vi "Serial-to-DTV_v1.vi"(10 "Input_U8":u8[](array[numeric])) -> (0 "mseg":u16, 2 "Data Validity Time":u16[](array[numeric]))   [LabVIEW 2017]
panel:
  out "seg":u8
  out "min":u8
  out "hora":u8
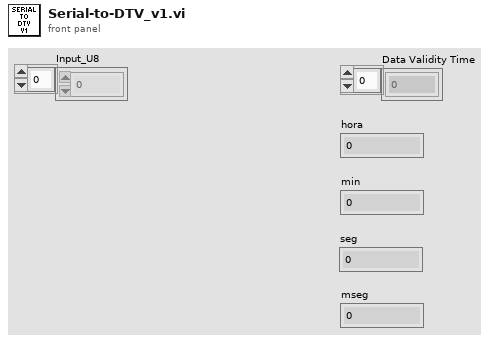
[diagram p1: front panel]
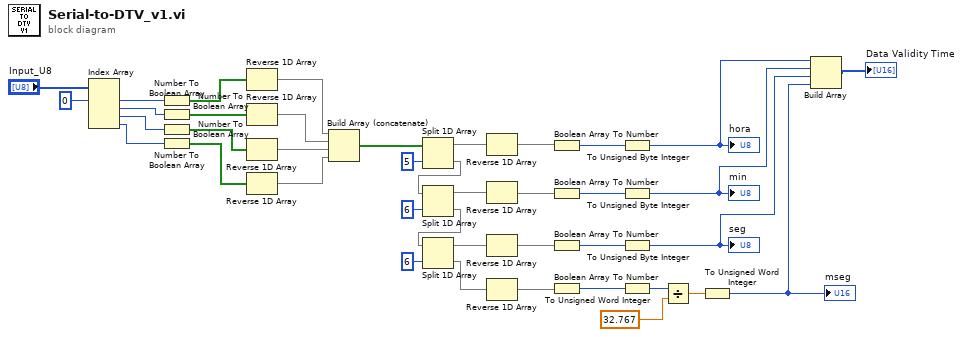
[diagram p0: block diagram]
diagram:
  n1 = Index Array(array="Input_U8", index #1=0 ("index")) -> (element #1=w36:u8, element #2=w37:u8, element #3=w38:u8, element #4=w39:u8)  [unwired: 3 in]
  n2 = Number To Boolean Array(number=w36) -> (Boolean array=w4:bool[])
  n3 = Number To Boolean Array(number=w37) -> (Boolean array=w3:bool[])
  n4 = Number To Boolean Array(number=w38) -> (Boolean array=w2:bool[])
  n5 = Number To Boolean Array(number=w39) -> (Boolean array=w1:bool[])
  n6 = Reverse 1D Array(array=w4) -> (reversed array=w33:bool[])
  n7 = Reverse 1D Array(array=w3) -> (reversed array=w32:bool[])
  n8 = Reverse 1D Array(array=w2) -> (reversed array=w31:bool[])
  n9 = Reverse 1D Array(array=w1) -> (reversed array=w30:bool[])
  n10 = Build Array (concatenate)(w33, w32, w31, w30) -> (w23:bool[])
  n11 = Split 1D Array(array=w23, index=5) -> (first subarray=w11:bool[], second subarray=w27:bool[])
  n12 = Split 1D Array(array=w27, index=6) -> (first subarray=w15:bool[], second subarray=w28:bool[])
  n13 = Split 1D Array(array=w28, index=6) -> (first subarray=w14:bool[], second subarray=w13:bool[])
  n14 = Reverse 1D Array(array=w11) -> (reversed array=w10:bool[])
  n15 = Reverse 1D Array(array=w15) -> (reversed array=w16:bool[])
  n16 = Reverse 1D Array(array=w14) -> (reversed array=w17:bool[])
  n17 = Reverse 1D Array(array=w13) -> (reversed array=w12:bool[])
  n18 = Boolean Array To Number(Boolean array=w10) -> (number=w20:u32)
  n19 = Boolean Array To Number(Boolean array=w16) -> (number=w19:u32)
  n20 = Boolean Array To Number(Boolean array=w17) -> (number=w18:u32)
  n21 = Boolean Array To Number(Boolean array=w12) -> (number=w22:u32)
  n22 = To Unsigned Byte Integer(number=w20) -> (unsigned 8bit integer=w5:u8)
  "hora" <- w5
  n23 = To Unsigned Byte Integer(number=w19) -> (unsigned 8bit integer=w6:u8)
  "min" <- w6
  n24 = To Unsigned Byte Integer(number=w18) -> (unsigned 8bit integer=w7:u8)
  "seg" <- w7
  n25 = To Unsigned Word Integer(number=w22) -> (unsigned 16bit integer=w21:u16)
  n26 = Divide(x=w21, y=32.767) -> (x/y=w9:dbl)
  n27 = To Unsigned Word Integer(number=w9) -> (unsigned 16bit integer=w8:u16)
  "mseg" <- w8
  n28 = Build Array(w5, w6, w7, w8) -> (→"Data Validity Time":u16[])
